vi "Write Joystick State Ref.vi"(8 "error in (no error)":errorcluster, 10 "Joystick State Ref":refnum<vi>, 11 "Test-XBox Controller-Receive Updates in":refnum<class "Test-XBox Controller-Receive Updates.lvclass">) -> (0 "error out":errorcluster, 3 "Test-XBox Controller-Receive Updates out":refnum<class "Test-XBox Controller-Receive Updates.lvclass">)   [LabVIEW 2014, in "Comp XBox One Controller.lvlib" / "Test-XBox Controller-Receive Updates.lvclass"]
uses:
  Test-XBox Controller-Receive Updates.lvclass
  Robot/Joystick/Joystick Class/Joystick State.ctl
  Robot/Joystick/Joystick Class/Button State.ctl
  Robot/Joystick/Joystick Class/Axis State.ctl
  Test-XBox Controller-Receive Updates.lvclass/Test-XBox Controller-Receive Updates.ctl
  Robot/Joystick/Joystick Class/Joystick.lvclass
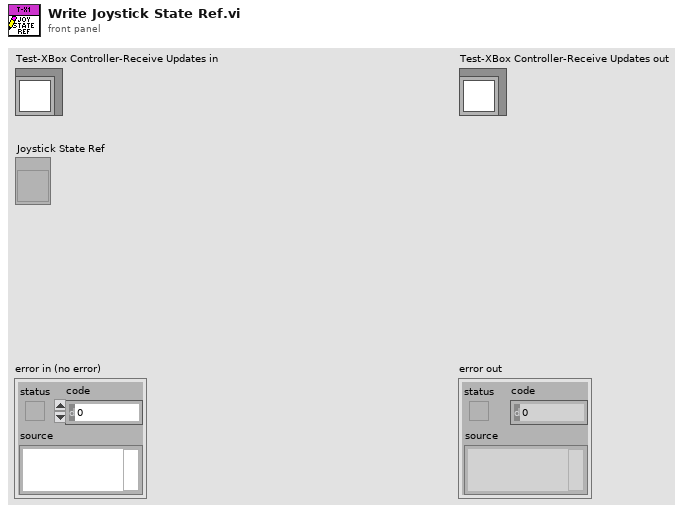
[diagram p1: front panel]
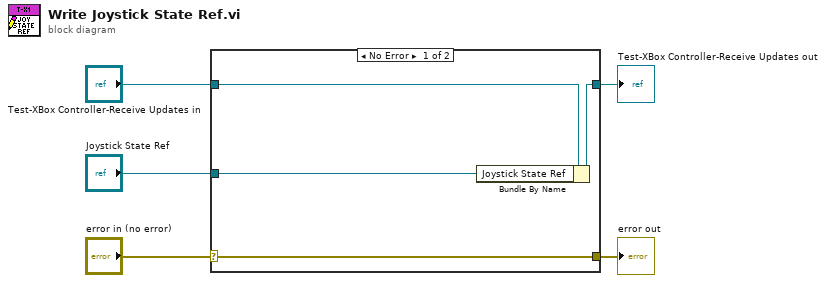
[diagram p0: block diagram]
diagram:
  n1 = case shown="No Error" "error in (no error)" {
    selector: "error in (no error)" -> [w9 w10]
    tunnel: [w9 w10] -> w4
    tunnel: [w7 w11] -> w2
    tunnel: "Test-XBox Controller-Receive Updates in" -> [w8 w11]
    tunnel: "Joystick State Ref" -> [w6 _]
    frame No Error {
      n2 = Bundle By Name(cluster=w8, "Joystick State Ref"=w6) -> (w7:refnum<class "Test-XBox Controller-Receive Updates.lvclass">)
    }
    frame Error {
    }
  }
  "error out" <- w4
  "Test-XBox Controller-Receive Updates out" <- w2
